vi "Processing Step.vi"(8 "error in (no error)":errorcluster, 11 "Controller Handler in":refnum<class "Controller Handler.lvclass">) -> (0 "error out":errorcluster, 2 "Processing Step":T1, 3 "Controller Handler out":refnum<class "Controller Handler.lvclass">)   [LabVIEW 2020, in "HTTP Server.lvlib" / "Controller Handler.lvclass"]
uses:
  Controller Handler.lvclass
  Processing Step.ctl
  HTTP Server.lvlib
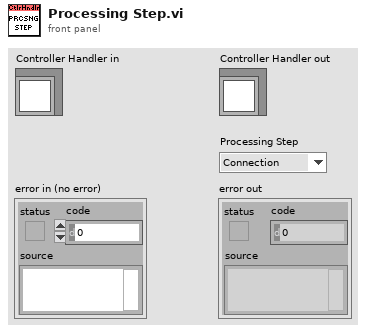
[diagram p1: front panel]
types:
  T1 = typedef "HTTP Server.lvlib/Processing Step.ctl" = enum16{"Connection", "Request", "Routing", "Controller Init", "Controller", "Response", "Cleanup", "Exception"}
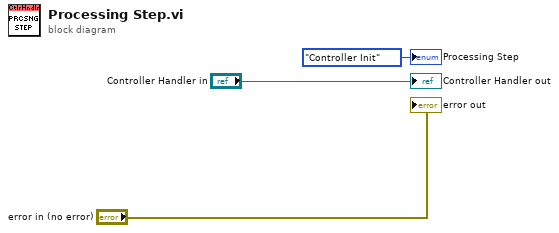
[diagram p0: block diagram]
diagram:
  "error out" <- "error in (no error)"
  "Controller Handler out" <- "Controller Handler in"
  "Processing Step" <- Processing_Step."Controller Init" ("Processing Step")
